vi "Timer.vi"(0 "Wait_Time":dbl=10.0 format="%#_13g", 11 "Error_In":errorcluster, 13 "Timer_Select":T1=enum."Time_Out?") -> (4 "Time_Out?":bool, 15 "Error_Out":errorcluster)   [LabVIEW 2023]
doc: "Used for time out opertion."
uses:
  Controls/Timer_Select.ctl
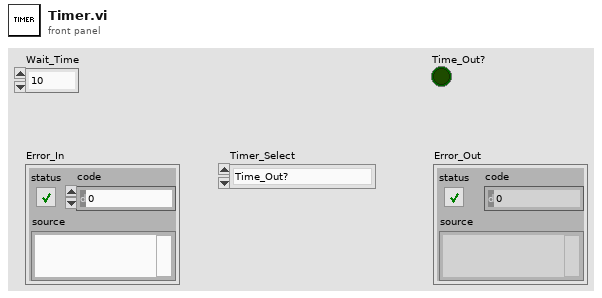
[diagram p1: front panel]
types:
  T1 = typedef "Timer_Select.ctl" = enum16{"Start_Timer", "Time_Out?", "Stop_Timer"}
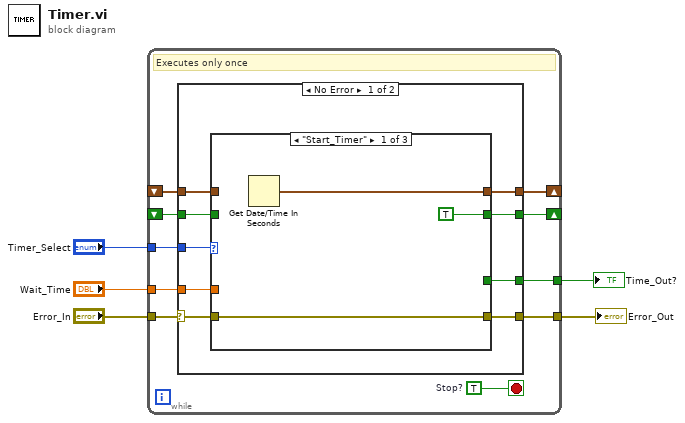
[diagram p0: block diagram]
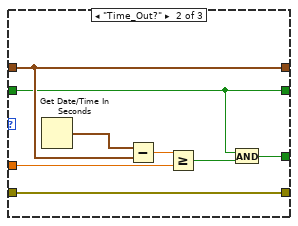
[diagram p2: hidden frame]
diagram:
  n1 = while {
    tunnel: "Timer_Select" -> [w15]
    shift-right: [w14] -> _
    shift-left: _ -> [w13]
    tunnel: [w12] -> w4
    tunnel: "Error_In" -> [w10]
    tunnel: [w9] -> w2
    shift-right: [w8] -> _
    shift-left: _ -> [w7]
    tunnel: "Wait_Time" -> [w6]
    stop <- w11 stop-if-true
    w11 = TRUE  # Stop?
    # "Executes only once"
    n2 = case shown="No Error" w10 {
      selector: w10 -> [w20 w37]
      tunnel: w15 -> [w24 _]
      tunnel: [w23 w38] -> w14
      tunnel: w13 -> [w22 w38]
      tunnel: [w21 _] -> w12
      tunnel: [w19 w37] -> w9
      tunnel: [w18 _] -> w8
      tunnel: w7 -> [w17 _]
      tunnel: w6 -> [w16 _]
      frame No Error {
        n3 = case shown="\"Start_Timer\"" w24 {
          tunnel: [w26 w35 _] -> w23
          tunnel: w22 -> [_ w35 _]
          tunnel: [_ w30 _] -> w21
          tunnel: w20 -> [w27 w32 w36]
          tunnel: [w27 w32 w36] -> w19
          tunnel: [TRUE w29 _] -> w18
          tunnel: w17 -> [_ w29 _]
          tunnel: w16 -> [_ w28 _]
          frame "Start_Timer" {
            n4 = Get Date/Time In Seconds() -> (seconds since 1Jan1904=w26:timestamp)
          }
          frame "Time_Out?" {
            n5 = Get Date/Time In Seconds() -> (seconds since 1Jan1904=w31:timestamp)
            n6 = Subtract(x=w31, y=w35) -> (x-y=w34:dbl)
            n7 = Greater Or Equal?(x=w34, y=w28) -> (x >= y?=w33:bool)
            n8 = And(x=w29, y=w33) -> (x .and. y?=w30:bool)
          }
          frame "Stop_Timer" {
          }
        }
      }
      frame Error {
      }
    }
  }
  "Time_Out?" <- w4
  "Error_Out" <- w2
